vi "PIDRelay.vi"(5 "setpoint":dbl format="%.2f", 6 "VISA resource name 2":refnum<visa-resource-name>, 7 "process variable":dbl format="%.2f") -> ()   [LabVIEW 2023]
uses:
  <vilib>/Instr/_visa.llb/VISA Configure Serial Port (Instr).vi
  <vilib>/addons/control/pid/NI_PID_autopid.lvlib
panel:
  out "tuning completed?":bool
  out "PID gains out":T1={"proportional gain (Kc)"=1.0, "integral time (Ti, min)"=0.01, "derivative time (Td, min)"=0.0} {"derivative time (Td, min)" format="%.3f"; "integral time (Ti, min)" format="%.3f"; "proportional gain (Kc)" format="%.3f"}
  in  "reinitialize? (F)":bool
  in  "autotuning parameters":T2={"controller type"=1, "relay cycles"=3, "relay amplitude"=1.0, "control specification"=2, "PV noise level"=0.1} {"PV noise level" format="%.2f"; "control specification" items=["normal", "fast", "slow"]; "relay amplitude" format="%.2f"; "controller type" items=["PID", "PI", "P"]}
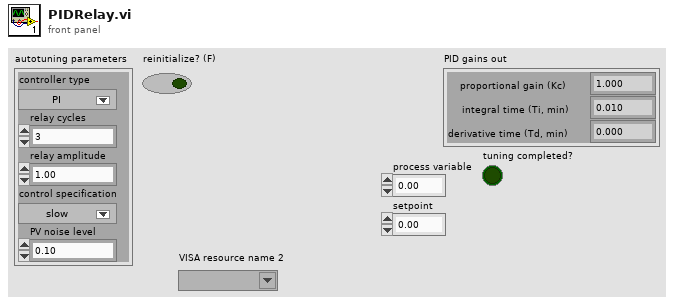
[diagram p1: front panel]
types:
  T1 = cluster{"proportional gain (Kc)":dbl, "integral time (Ti, min)":dbl, "derivative time (Td, min)":dbl}
  T2 = cluster{"controller type":u16, "relay cycles":i32, "relay amplitude":dbl, "control specification":u16, "PV noise level":dbl}
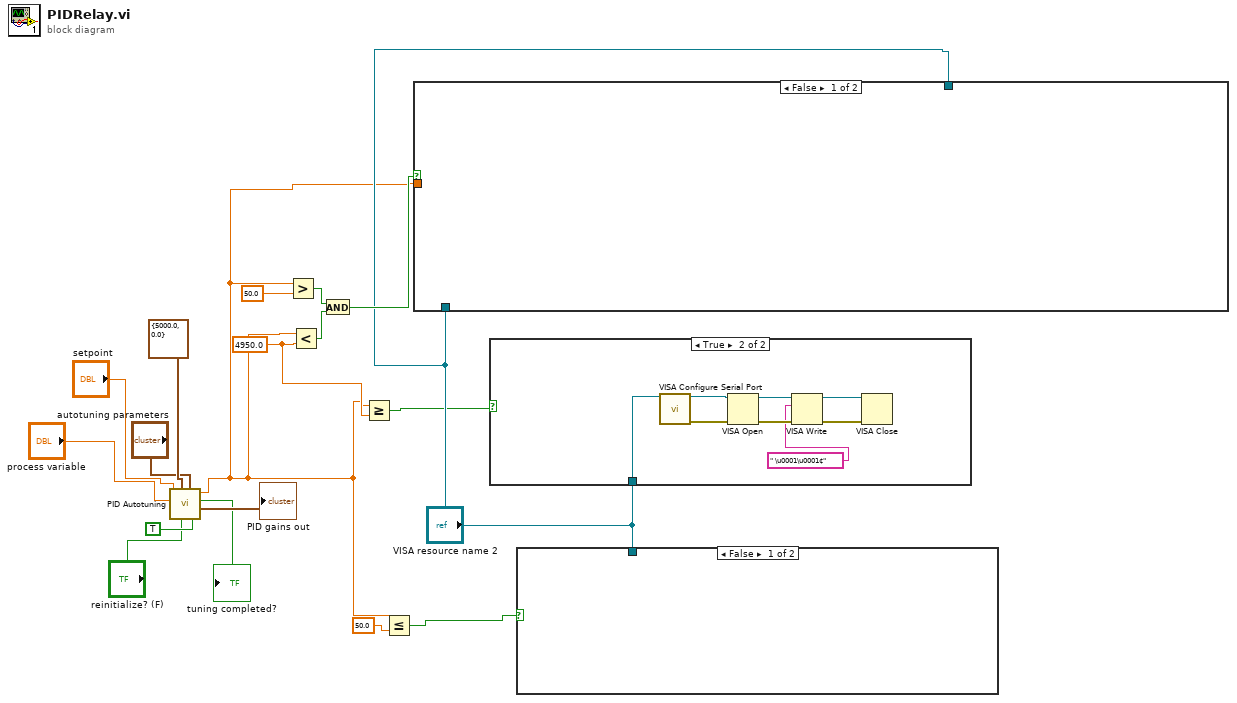
[diagram p0: block diagram]
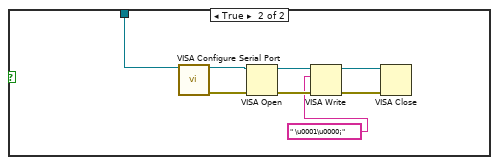
[diagram p2: hidden frame]
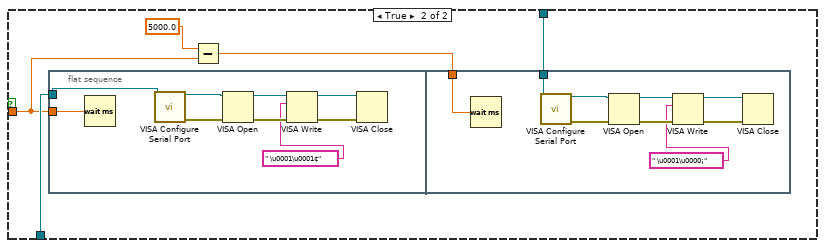
[diagram p3: hidden frame]
diagram:
  w12 = 4950.0 ("y")
  n1 = call <vilib>:"PID Autotuning.vi"("autotune? (F)"=TRUE ("reinitialize? (F)"), "autotuning parameters"="autotuning parameters", "reinitialize? (F)"="reinitialize? (F)", "output range"=cluster{"output high":dbl, "output low":dbl} {"output high"=5000.0, "output low"=0.0}, "process variable"="process variable", "setpoint"="setpoint") -> ("PID gains out"=→"PID gains out":T1, "tuning completed?"=→"tuning completed?":bool, "output"=w9:dbl)  [unwired: 2 in, 1 out]
  n2 = Greater?(x=w9, y=50.0) -> (0:w15:bool)
  n3 = Less?(x=w9, y=w12) -> (x < y?=w14:bool)
  n4 = And(x=w15, y=w14) -> (x .and. y?=w18:bool)
  n5 = Greater Or Equal?(x=w9, y=w12) -> (x >= y?=w13:bool)
  n6 = Less Or Equal?(x=w9, y=50.0) -> (x <= y?=w10:bool)
  n7 = case shown="False" w18 {
    tunnel: "VISA resource name 2" -> [_ w23]
    tunnel: "VISA resource name 2" -> [_ w22]
    tunnel: w9 -> [_ w19]
    frame False {
    }
    frame True {
      n8 = flat-sequence {
        tunnel: w23 -> [w25]
        tunnel: w19 -> [w24]
        tunnel: w22 -> [w34]
        tunnel: w21 -> [w33]
        frame #0 {
          n9 = Wait (ms)(milliseconds to wait=w24) -> ()  [unwired: 1 out]
          n10 = call-poly "VISA Configure Serial Port"("VISA resource name"=w25) -> ("VISA resource name out"=w32:refnum<visa-resource-name>, "error out"=w31:errorcluster)  [unwired: 13 in]
          n11 = VISA Open(error in (no error)=w31, VISA resource name=w32) -> (VISA resource name=w30:refnum<visa-resource-name>, error out=w29:errorcluster)  [unwired: 3 in]
          n12 = VISA Write(VISA resource name=w30, write buffer=" \u0001\u0001¢", error in (no error)=w29) -> (VISA resource name out=w28:refnum<visa-resource-name>, error out=w27:errorcluster)  [unwired: 1 out]
          n13 = VISA Close(VISA resource name=w28, error in (no error)=w27) -> ()  [unwired: 1 out]
        }
        frame #1 {
          n14 = Wait (ms)(milliseconds to wait=w33) -> ()  [unwired: 1 out]
          n15 = call-poly "VISA Configure Serial Port"("VISA resource name"=w34) -> ("VISA resource name out"=w36:refnum<visa-resource-name>, "error out"=w37:errorcluster)  [unwired: 13 in]
          n16 = VISA Open(error in (no error)=w37, VISA resource name=w36) -> (VISA resource name=w38:refnum<visa-resource-name>, error out=w39:errorcluster)  [unwired: 3 in]
          n17 = VISA Write(VISA resource name=w38, write buffer=" \u0001\u0000¡", error in (no error)=w39) -> (VISA resource name out=w40:refnum<visa-resource-name>, error out=w41:errorcluster)  [unwired: 1 out]
          n18 = VISA Close(VISA resource name=w40, error in (no error)=w41) -> ()  [unwired: 1 out]
        }
      }
      n19 = Subtract(x=5000.0, y=w19) -> (x-y=w21:dbl)
    }
  }
  n20 = case shown="True" w13 {
    tunnel: "VISA resource name 2" -> [_ w42]
    frame False {
    }
    frame True {
      n21 = call-poly "VISA Configure Serial Port"("VISA resource name"=w42) -> ("VISA resource name out"=w49:refnum<visa-resource-name>, "error out"=w48:errorcluster)  [unwired: 13 in]
      n22 = VISA Open(error in (no error)=w48, VISA resource name=w49) -> (VISA resource name=w47:refnum<visa-resource-name>, error out=w46:errorcluster)  [unwired: 3 in]
      n23 = VISA Write(VISA resource name=w47, write buffer=" \u0001\u0001¢", error in (no error)=w46) -> (VISA resource name out=w45:refnum<visa-resource-name>, error out=w44:errorcluster)  [unwired: 1 out]
      n24 = VISA Close(VISA resource name=w45, error in (no error)=w44) -> ()  [unwired: 1 out]
    }
  }
  n25 = case shown="False" w10 {
    tunnel: "VISA resource name 2" -> [_ w50]
    frame False {
    }
    frame True {
      n26 = call-poly "VISA Configure Serial Port"("VISA resource name"=w50) -> ("VISA resource name out"=w57:refnum<visa-resource-name>, "error out"=w56:errorcluster)  [unwired: 13 in]
      n27 = VISA Open(error in (no error)=w56, VISA resource name=w57) -> (VISA resource name=w55:refnum<visa-resource-name>, error out=w54:errorcluster)  [unwired: 3 in]
      n28 = VISA Write(VISA resource name=w55, write buffer=" \u0001\u0000¡", error in (no error)=w54) -> (VISA resource name out=w53:refnum<visa-resource-name>, error out=w52:errorcluster)  [unwired: 1 out]
      n29 = VISA Close(VISA resource name=w53, error in (no error)=w52) -> ()  [unwired: 1 out]
    }
  }
